vi "Export VI ConPane.vi"() -> ()   [LabVIEW 2021]
panel:
  out "Error":errorcluster
  in  "Images Dir":path=path "C:/Projects/LabVIEW/RyLibs/ry.lib/ryTimer/Help/Images"
  in  "VI Path":path
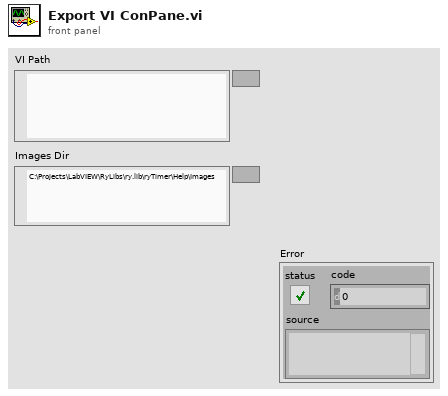
[diagram p1: front panel]
types:
  T1 = typedef "imagedata.ctl" = cluster{"image type":i32, "image depth":i32, "image":u8[], "mask":u8[], "colors":u32[], "Rectangle":cluster{"left":i16, "top":i16, "right":i16, "bottom":i16}}
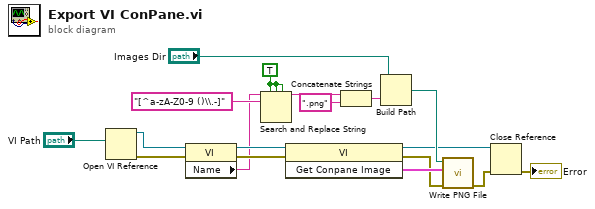
[diagram p0: block diagram]
diagram:
  w14 = TRUE ("replace all? (F)")
  n1 = Open VI Reference(vi path="VI Path") -> (vi reference=w7:refnum<vi>, error out=w17:errorcluster)  [unwired: 5 in]
  n2 = property class="VI"(reference=w7, error in=w17) -> (reference out=w6:refnum<vi>, error out=w8:errorcluster, "Name"=w5:string)
  n3 = Search and Replace String(replace all?=w14, case sensitive?=w14, multiline?=w14, input string=w5, search string="[^a-zA-Z0-9 ()\\.-]") -> (result string=w12:string)  [unwired: 3 in, 3 out]
  n4 = invoke class="VI" method="Get Conpane Image"(reference=w6, error in=w8) -> (reference out=w2:refnum<vi>, error out=w15:errorcluster, "Get Conpane Image"=w16:T1)  [unwired: 1 in]
  n5 = Concatenate Strings(w12, ".png" ("string")) -> (w11:string)
  n6 = Build Path(base path="Images Dir", name or relative path=w11) -> (appended path=w4:path)
  n7 = call <vilib>:"Write PNG File.vi"("error in (no error)"=w15, "image data"=w16, "path to PNG file"=w4) -> ("error out"=w3:errorcluster)  [unwired: 7 in, 1 out]
  n8 = Close Reference(reference=w2, error in (no error)=w3) -> (error out=→"Error":errorcluster)
